vi "TypeDescriptor_DescriptorElementsToVariantCluster.vi"(9 "Data String":string, 11 "type descriptor":i16[](array[numeric]) format="%04x") -> (0 "concatenated element descriptors":i16[](array[numeric]), 1 "Nb elements":i32, 2 "elements":T1[](array[typedef]), 3 "type descriptor dup":i16[](array[numeric]) format="%.0x")   [LabVIEW 2013]
uses:
  OpenDescriptor -- cluster.ctl
  TypeDescriptor_GetPString.vi
  OpenDescriptor.lvlib
  Conversions/OpenConvert.lvlib
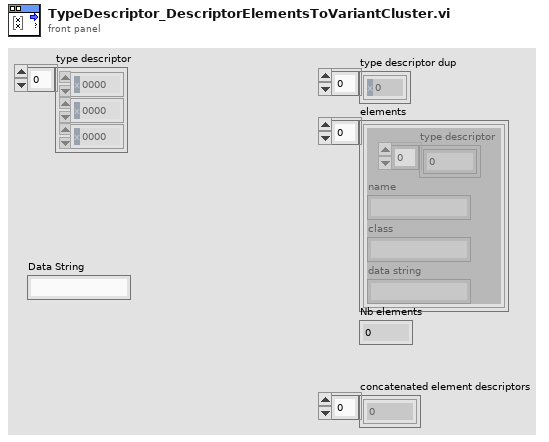
[diagram p1: front panel]
types:
  T1 = typedef "OpenDescriptor.lvlib/OpenDescriptor -- cluster.ctl" = cluster{"type descriptor":i16[], "name":string, "class":string, "data string":string}
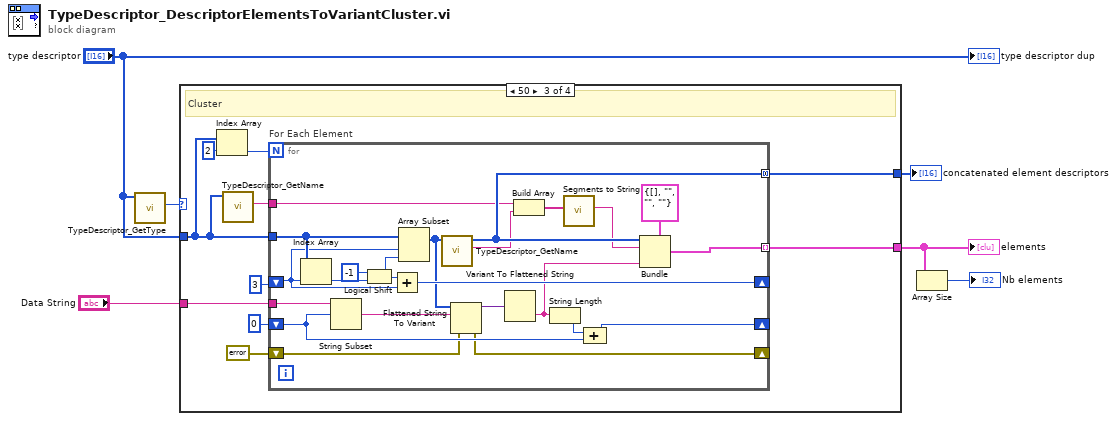
[diagram p0: block diagram]
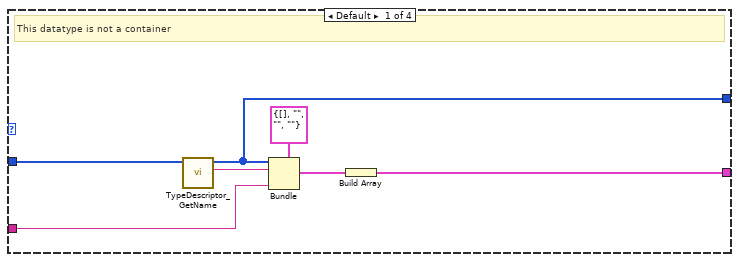
[diagram p2: hidden frame]
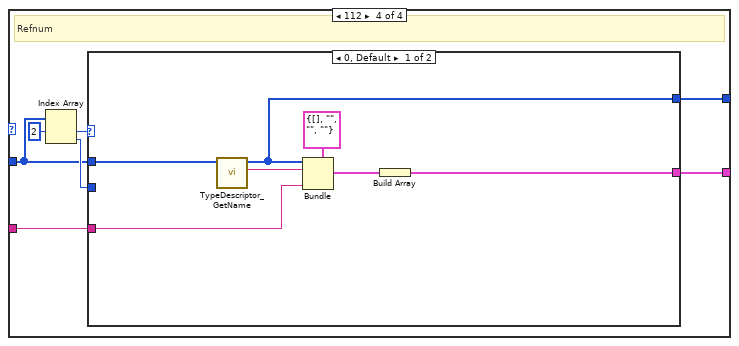
[diagram p4: hidden frame]
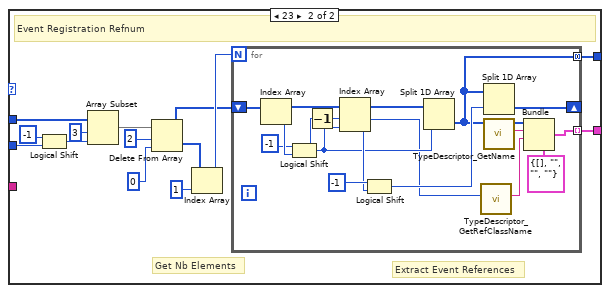
[diagram p5: hidden frame]
diagram:
  n1 = call "TypeDescriptor_GetType.vi"("type descriptor"="type descriptor") -> ("Type"=w5:u8)  [unwired: 9 in, 1 out]
  n2 = case shown="50" w5 {
    tunnel: [w9 _ w20 w49] -> w4
    tunnel: "type descriptor" -> [w11 _ w15 w50]
    tunnel: [w8 _ w19 w48] -> w2
    tunnel: "Data String" -> [w7 _ w17 w47]
    frame Default {
      # "This datatype is not a container"
      n3 = call "TypeDescriptor_GetName.vi"("type descriptor"=w11) -> ("name"=w13:string, "type descriptor dup"=w8:i16[])  [unwired: 8 in, 1 out]
      n4 = Bundle(cluster=T1 {"type descriptor"=[], "name"="", "class"="", "data string"=""} ("Descriptor Element"), "type descriptor"=w8, "name"=w13, "data string"=w7) -> (w10:T1)  [unwired: 1 in]
      n5 = Build Array(w10) -> (w9:T1[])
    }
    frame 0 {
      # "void"
    }
    frame 80 {
      # "Cluster"
      n6 = Index Array(array=w15, index=2) -> (element=w22:i16)
      n7 = call "TypeDescriptor_GetName.vi"("type descriptor"=w15) -> ("name"=w14:string)  [unwired: 8 in, 2 out]
      n8 = for "For Each Element" {
        N: w22 -> [_]
        tunnel: w15 -> [w43]
        shift-right: [w44] -> _
        shift-left: 3 ("index") -> [w42]
        tunnel: [w40] -> w20 mode=indexing
        tunnel: [w38] -> w19 mode=concatenating
        shift-right: [w31] -> _
        shift-left: 0 -> [w32]
        tunnel: w17 -> [w37]
        shift-right: [w28] -> _
        shift-left: errorcluster {"status"=FALSE, "code"=0, "source"=""} ("error out") -> [w29]
        tunnel: w14 -> [w27]
        n9 = Index Array(array=w43, index=w42) -> (element=w45:i16)
        n10 = String Subset(string=w37, offset (0)=w32) -> (substring=w35:string)  [unwired: 1 in]
        n11 = Logical Shift(y=i16 -1, x=w45) -> (x << y=w41:i16)
        n12 = Add(x=w41, y=w42) -> (x+y=w44:i32)
        n13 = Array Subset(array=w43, index=w42, length=w41) -> (w36:i16[])
        n14 = call "TypeDescriptor_GetName.vi"("type descriptor"=w36) -> ("name"=w25:string, "type descriptor dup"=w38:i16[])  [unwired: 8 in, 1 out]
        n15 = Flattened String To Variant(4:w29, 6:w35, 7:w36) -> (0:w28:errorcluster, 3:w34:variant)
        n16 = Variant To Flattened String(Variant=w34) -> (data string=w30:string)  [unwired: 1 out]
        n17 = Build Array(w27, w25) -> (w26:string[])
        n18 = String Length(string=w30) -> (length=w33:i32)
        n19 = call "Segments to String.vi"("Segments"=w26) -> ("String"=w24:string)  [unwired: 10 in]
        n20 = Compound Arithmetic op=ADD(w33, w32) -> (w31:i32)
        n21 = Bundle(cluster=T1 {"type descriptor"=[], "name"="", "class"="", "data string"=""} ("Descriptor Element"), "type descriptor"=w38, "name"=w24, "data string"=w30) -> (w40:T1)  [unwired: 1 in]
      }
    }
    frame 112 {
      # "Refnum"
      n22 = Index Array(array=w50, index #1=2 ("index")) -> (element #1=w52:i16, element #2=w51:i16)  [unwired: 1 in]
      n23 = case shown="0, Default" w52 {
        tunnel: w51 -> [_ w71]
        tunnel: w50 -> [w57 w74]
        tunnel: [w55 w62] -> w49
        tunnel: [w56 w61] -> w48
        tunnel: w47 -> [w54 _]
        frame 0, Default {
          n24 = call "TypeDescriptor_GetName.vi"("type descriptor"=w57) -> ("name"=w58:string, "type descriptor dup"=w56:i16[])  [unwired: 8 in, 1 out]
          n25 = Bundle(cluster=T1 {"type descriptor"=[], "name"="", "class"="", "data string"=""} ("Descriptor Element"), "type descriptor"=w56, "name"=w58, "data string"=w54) -> (w60:T1)  [unwired: 1 in]
          n26 = Build Array(w60) -> (w55:T1[])
        }
        frame 23 {
          # "Extract Event References"
          # "Get Nb Elements"
          # "Event Registration Refnum"
          n27 = Logical Shift(y=i16 -1, x=w71) -> (x << y=w70:i16)
          n28 = Array Subset(array=w74, index=3, length=w70) -> (w69:i16[])
          n29 = Delete From Array(array=w69, length=2 ("index"), index=0) -> (deleted portion=w67:i16[], array with subset deleted=w63:i16[])
          n30 = Index Array(array=w67, index=1) -> (element=w64:i16)
          n31 = for {
            N: w64 -> [_]
            shift-right: [w82] -> _
            shift-left: w63 -> [w85]
            tunnel: [w77] -> w62 mode=indexing
            tunnel: [w75] -> w61 mode=concatenating
            n32 = Index Array(array=w85) -> (element=w90:i16)  [unwired: 1 in]
            n33 = Logical Shift(y=i16 -1, x=w90) -> (x << y=w84:i16)
            n34 = Decrement(x=w84) -> (x-1=w86:i16)
            n35 = Index Array(array=w85, index #1=w86, index #2=w84) -> (element #1=w81:i16, element #2=w87:i16)
            n36 = Logical Shift(y=i16 -1, x=w87) -> (x << y=w83:i16)
            n37 = Split 1D Array(array=w85, index=w84) -> (second subarray=w75:i16[])  [unwired: 1 out]
            n38 = call "TypeDescriptor_GetRefClassName.vi"("Ref Class"=w81) -> ("Reference Class"=w79:string)  [unwired: 10 in]
            n39 = Split 1D Array(array=w75, index=w83) -> (second subarray=w82:i16[])  [unwired: 1 out]
            n40 = call "TypeDescriptor_GetName.vi"("type descriptor"=w75) -> ("name"=w78:string, "type descriptor dup"=w80:i16[])  [unwired: 8 in, 1 out]
            n41 = Bundle(cluster=T1 {"type descriptor"=[], "name"="", "class"="", "data string"=""} ("Descriptor Element"), "type descriptor"=w80, "name"=w78, "class"=w79) -> (w77:T1)  [unwired: 1 in]
          }
        }
      }
    }
  }
  "elements" <- w4
  "concatenated element descriptors" <- w2
  n42 = Array Size(array=w4) -> (size(s)=→"Nb elements":i32)
  "type descriptor dup" <- "type descriptor"
